vi "server app properties.vi"(8 "error in (no error)":errorcluster) -> (0 "error out":errorcluster, 2 "App.AllVIs":string[](array[string]), 3 "App.Properties":T1)   [LabVIEW 2011]
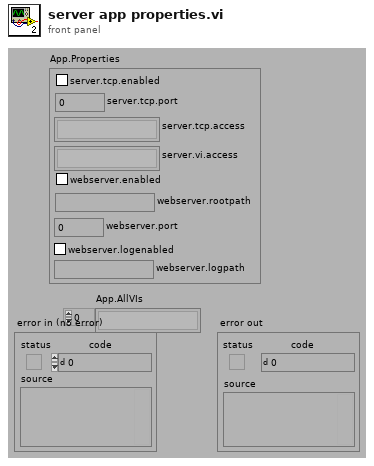
[diagram p1: front panel]
types:
  T1 = cluster{"webserver.rootpath":path, "server.tcp.enabled":bool, "server.tcp.port":u32, "server.tcp.access":string[], "server.vi.access":string[], "webserver.enabled":bool, "webserver.port":u16, "webserver.logenabled":bool, "webserver.logpath":path}
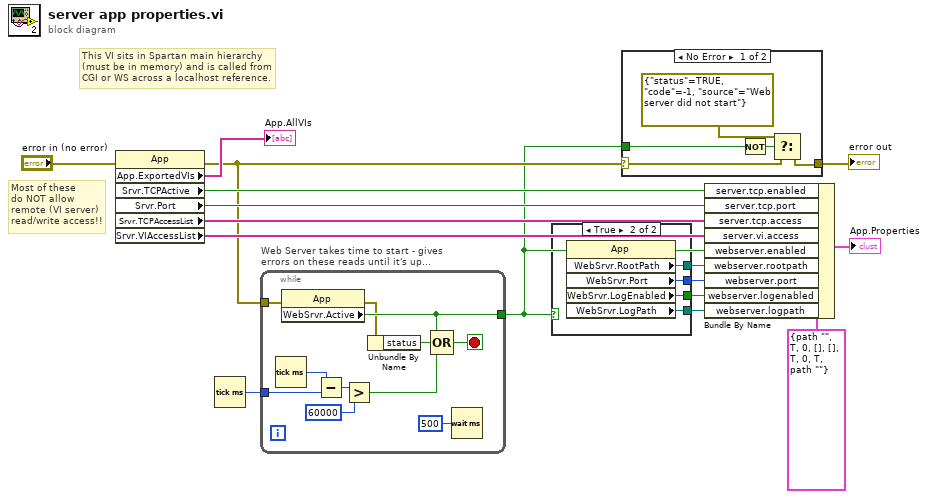
[diagram p0: block diagram]
diagram:
  # "Most of these\ndo NOT allow\nremote (VI server)\nread/write access!!"
  # "This VI sits in Spartan main hierarchy\n(must be in memory) and is called from\nCGI or WS across a localhost reference."
  n1 = property class="App"(error in="error in (no error)") -> (error out=w7:errorcluster, "App.ExportedVIs"=→"App.AllVIs":string[], "Srvr.TCPActive"=w15:bool, "Srvr.Port"=w14:u32, "Srvr.TCPAccessList"=w13:string[], "Srvr.VIAccessList"=w12:string[])  [unwired: 1 in, 1 out]
  n2 = Tick Count (ms)() -> (millisecond timer value=w8:u32)
  n3 = while "Web Server takes time to start - gives\nerrors on these reads until it's up..." {
    tunnel: w7 -> [w19]
    tunnel: w8 -> [w26]
    tunnel: [w18] -> w5
    stop <- w21 stop-if-true
    n4 = Tick Count (ms)() -> (millisecond timer value=w27:u32)
    n5 = property class="App"(error in=w19) -> (error out=w17:errorcluster, "WebSrvr.Active"=w18:bool)  [unwired: 1 in, 1 out]
    n6 = Subtract(x=w27, y=w26) -> (x-y=w25:u32)
    n7 = Greater?(x=w25, y=u32 60000) -> (0:w22:bool)
    n8 = Unbundle By Name(w17) -> ("status"=w23:bool)
    n9 = Compound Arithmetic op=OR(w18, w23, w22) -> (w21:bool)
    n10 = Wait (ms)(milliseconds to wait=u32 500) -> ()  [unwired: 1 out]
  }
  n11 = case shown="True" w5 {
    tunnel: [_ w31] -> w4
    tunnel: [_ w30] -> w3
    tunnel: [_ w29] -> w2
    tunnel: [_ w28] -> w1
    frame False {
    }
    frame True {
      n12 = property class="App"() -> ("WebSrvr.RootPath"=w31:path, "WebSrvr.Port"=w30:u16, "WebSrvr.LogEnabled"=w29:bool, "WebSrvr.LogPath"=w28:path)  [unwired: 2 in, 2 out]
    }
  }
  n13 = case shown="No Error" w7 {
    selector: w7 -> [w34 w37]
    tunnel: w5 -> [w36 _]
    tunnel: [w33 w37] -> w6
    frame No Error {
      n14 = Not(x=w36) -> (.not. x?=w35:bool)
      n15 = Select(t=errorcluster {"status"=TRUE, "code"=-1, "source"="Web server did not start"}, s=w35, f=w34) -> (s? t:f=w33:errorcluster)
    }
    frame Error {
    }
  }
  "error out" <- w6
  n16 = Bundle By Name(cluster=T1 {"webserver.rootpath"=path "", "server.tcp.enabled"=TRUE, "server.tcp.port"=0, "server.tcp.access"=[], "server.vi.access"=[], "webserver.enabled"=TRUE, "webserver.port"=0, "webserver.logenabled"=TRUE, "webserver.logpath"=path ""} ("App.Properties"), "server.tcp.enabled"=w15, "server.tcp.port"=w14, "server.tcp.access"=w13, "server.vi.access"=w12, "webserver.enabled"=w5, "webserver.rootpath"=w4, "webserver.port"=w3, "webserver.logenabled"=w2, "webserver.logpath"=w1) -> (→"App.Properties":T1)
